vi "Write State.vi"(10 "State":T1, 11 "Interlock in":refnum<class "Interlock.lvclass">) -> (3 "Interlock out":refnum<class "Interlock.lvclass">)   [LabVIEW 2015, in "Interlocks.lvlib" / "Interlock.lvclass"]
uses:
  Interlock.lvclass
  State Enum.ctl
  Interlock.lvclass/Interlock.ctl
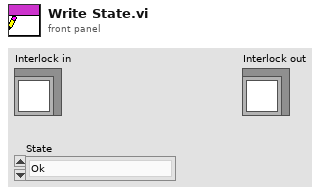
[diagram p1: front panel]
types:
  T1 = typedef "Interlocks.lvlib/Interlock.lvclass/State Enum.ctl" = enum16{"Ok", "Error", "Interlock", "Out of Range", "Is ON", "Is OFF", "Denied", "Not Allowed", "Sample Allow", "Sample Deny"}
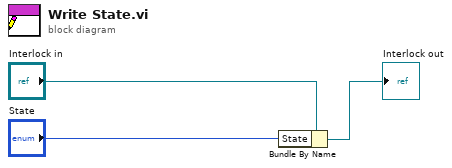
[diagram p0: block diagram]
diagram:
  n1 = Bundle By Name(cluster="Interlock in", "State"="State") -> (→"Interlock out":refnum<class "Interlock.lvclass">)
